vi "REPORT_AUDIT_define_scope_page.vi"(7 "active_page":i32, 9 "records":string[][](array[string]), 10 "amount_record":i32, 11 "ids":string[](array[string])) -> (2 "size":i32, 3 "start_row":i32)   [LabVIEW 2020]
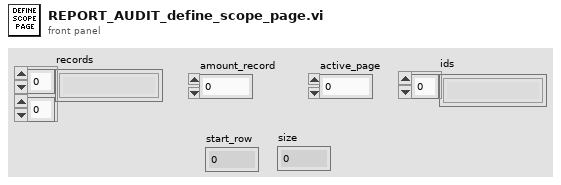
[diagram p1: front panel]
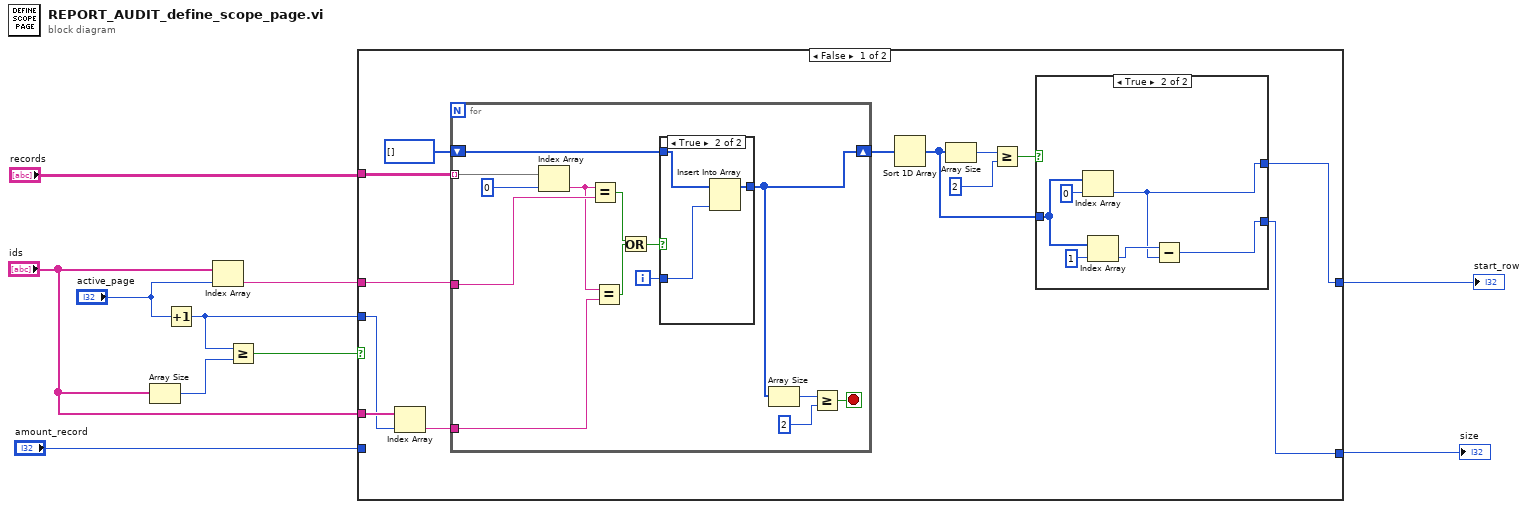
[diagram p0: block diagram]
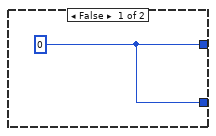
[diagram p2: hidden frame]
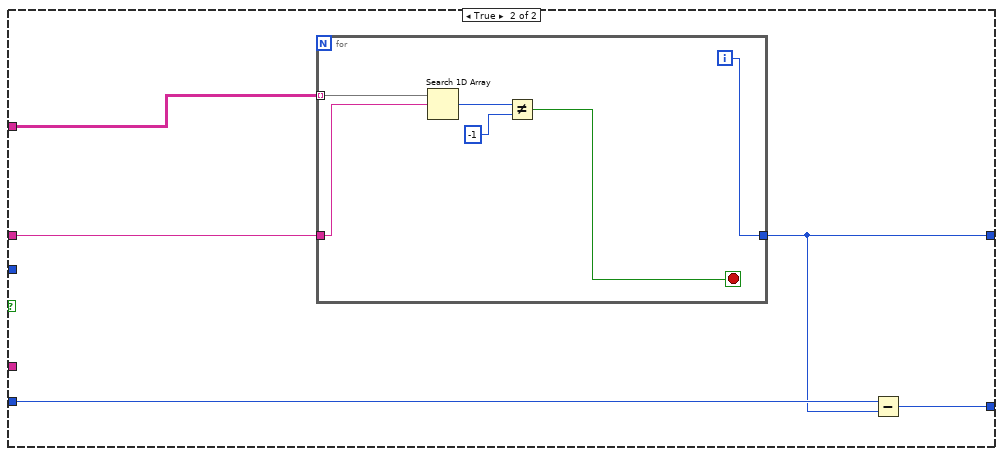
[diagram p4: hidden frame]
diagram:
  n1 = Array Size(array="ids") -> (size(s)=w9:i32)
  n2 = Increment(x="active_page") -> (x+1=w4:i32)
  n3 = Index Array(array="ids", index="active_page") -> (element=w7:string)
  n4 = Greater Or Equal?(x=w4, y=w9) -> (x >= y?=w8:bool)
  n5 = case shown="False" w8 {
    tunnel: w7 -> [w20 w52]
    tunnel: "amount_record" -> [_ w51]
    tunnel: [w12 w50] -> w1
    tunnel: [w11 w49] -> w6
    tunnel: "ids" -> [w23 _]
    tunnel: w4 -> [w22 _]
    tunnel: "records" -> [w21 w53]
    frame False {
      n6 = Index Array(array=w23, index=w22) -> (element=w19:string)
      n7 = for {
        tunnel: w21 -> [w44] mode=indexing
        tunnel: w20 -> [w42]
        tunnel: w19 -> [w40]
        shift-right: [w34] -> w17
        shift-left: i32[] [] -> [w35]
        i -> [w36]
        stop <- w31 stop-if-true
        n8 = Index Array(array=w44, index=0) -> (element=w41:string)
        n9 = Equal?(x=w41, y=w42) -> (x = y?=w39:bool)
        n10 = Equal?(x=w41, y=w40) -> (x = y?=w38:bool)
        n11 = Or(x=w39, y=w38) -> (x .or. y?=w37:bool)
        n12 = case shown="True" w37 {
          tunnel: w36 -> [_ w48]
          tunnel: w35 -> [w45 w47]
          tunnel: [w45 w46] -> w34
          frame False {
          }
          frame True {
            n13 = Insert Into Array(array=w47, new element=w48) -> (w46:i32[])  [unwired: 1 in]
          }
        }
        n14 = Array Size(array=w34) -> (size(s)=w33:i32)
        n15 = Greater Or Equal?(x=w33, y=2) -> (x >= y?=w31:bool)
      }
      n16 = Sort 1D Array(array=w17) -> (sorted array=w13:i32[])
      n17 = Array Size(array=w13) -> (size(s)=w16:i32)
      n18 = Greater Or Equal?(x=w16, y=2) -> (x >= y?=w14:bool)
      n19 = case shown="True" w14 {
        tunnel: [w24 w26] -> w12
        tunnel: w13 -> [_ w28]
        tunnel: [w24 w25] -> w11
        frame False {
          w24 = 0
        }
        frame True {
          n20 = Index Array(array=w28, index=0) -> (element=w26:i32)
          n21 = Index Array(array=w28, index=1) -> (element=w27:i32)
          n22 = Subtract(x=w27, y=w26) -> (x-y=w25:i32)
        }
      }
    }
    frame True {
      n23 = for {
        tunnel: w53 -> [w59] mode=indexing
        tunnel: w52 -> [w58]
        tunnel: [w54] -> w50
        i -> [w54]
        stop <- w55 stop-if-true
        n24 = Search 1D Array(1D array=w59, element=w58) -> (index of element=w57:i32)  [unwired: 1 in]
        n25 = Not Equal?(x=w57, y=-1) -> (x != y?=w55:bool)
      }
      n26 = Subtract(x=w51, y=w50) -> (x-y=w49:i32)
    }
  }
  "start_row" <- w1
  "size" <- w6
